vi "Entradas.vi"(11 "Class 2.lvclass":refnum<class "Class 2.lvclass">) -> (3 "Class 2.lvclass 2":refnum<class "Class 2.lvclass">)   [LabVIEW 2019, in "Class 2.lvclass"]
uses:
  Class 2.lvclass
  Class 2.lvclass/Class 2.ctl
  Datos Out.vi
  Datos In.vi
panel:
  out "current time":u32
  out "current time 2":u32
  in  "PRUEBA DE CONTACTOS":string(combo)
  in  "PRUEBA DE DISTANCIA":string(combo)
  in  "PRUEBA DE TENSION":string(combo)
  in  "ENTRADAS.HOME C2":bool
  in  "ENTRADAS.PIEZA EN EL NIDO":bool
  in  "ENTRADAS.SMAC TOMA DE MUESTRA":bool
  in  "ENTRADAS.SMAC APROXIMACION":bool
  in  "ENTRADAS.SMAC AVANCE SEGURO":bool
  in  "ENTRADAS.SMAC HOME":bool
  in  "ENTRADAS.AVANCE C2":bool
  in  "ENTRADAS.AVANCE C1":bool
  in  "ENTRADAS.HOME C1":bool
  in  "ENTRADAS.BIMANUAL 2":bool
  in  "ENTRADAS.BIMANUAL 1":bool
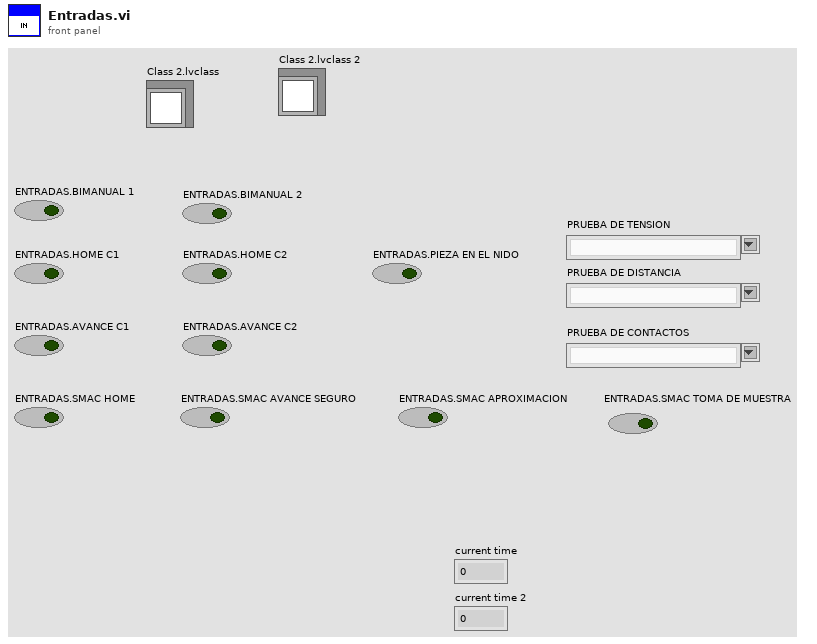
[diagram p1: front panel]
types:
  T1 = cluster{"Test":bool, "CILINDRO _1":bool, "CILINDRO _2":bool, "SMAC_RETORNANDO":bool, "SMAC_AVANZANDO":bool, "MANUAL":bool, "EST_1":bool, "EST_2":bool, "EST_3":bool, "MOVER A ORIGEN":bool, "RESET":bool, "PARO":bool, "INICIO":bool, "DATA_CONTROL":cluster{"ESTACION_1":cluster{"ACEPTADA":bool, "MAXIMO":dbl, "MINIMO":dbl, "LECTURA":dbl}, "ESTACION_2":cluster{"ACEPTADA":bool, "MAXIMO":dbl, "MINIMO":dbl, "LECTURA":dbl}, "ESTACION_3":cluster{"ACEPTADA":bool, "MAXIMO":dbl, "MINIMO":dbl, "LECTURA":dbl}}, "INGENIERIA O PROCESO":bool}
  T2 = cluster{"SALIDAS.CILINDRO 1":bool, "SALIDAS.CILINDRO 2":bool, "SALIDAS.SEMAC RETORNANDO":bool, "SALIDAS.SAMAC AVANZANDO":bool, "Auto(off)/Manual(on)":bool, "HOME_CILINDRO_1":bool, "HOME_CILINDRO_2":bool, "AVANCE_CILINDRO_1":bool, "AVANCE_CILINDRO_2":bool, "PIEZA_EN_NIDO":bool, "BIMANUAL 2":bool, "BIMANUAL1":bool, "SIN CAMBIOS":bool, "CON  CAMBIOS":bool, "TESTER":bool, "MAQUINA EN ORIGEN":bool, "FALLA PRESENTE":bool}
  T3 = cluster{"DATO GAP":string, "DATO TENSION":string, "mensajes usuario":string}
  T4 = cluster{"Numeric":dbl, "VALOR DE DISTANCIA":dbl, "VALOR DE TENSION":dbl}
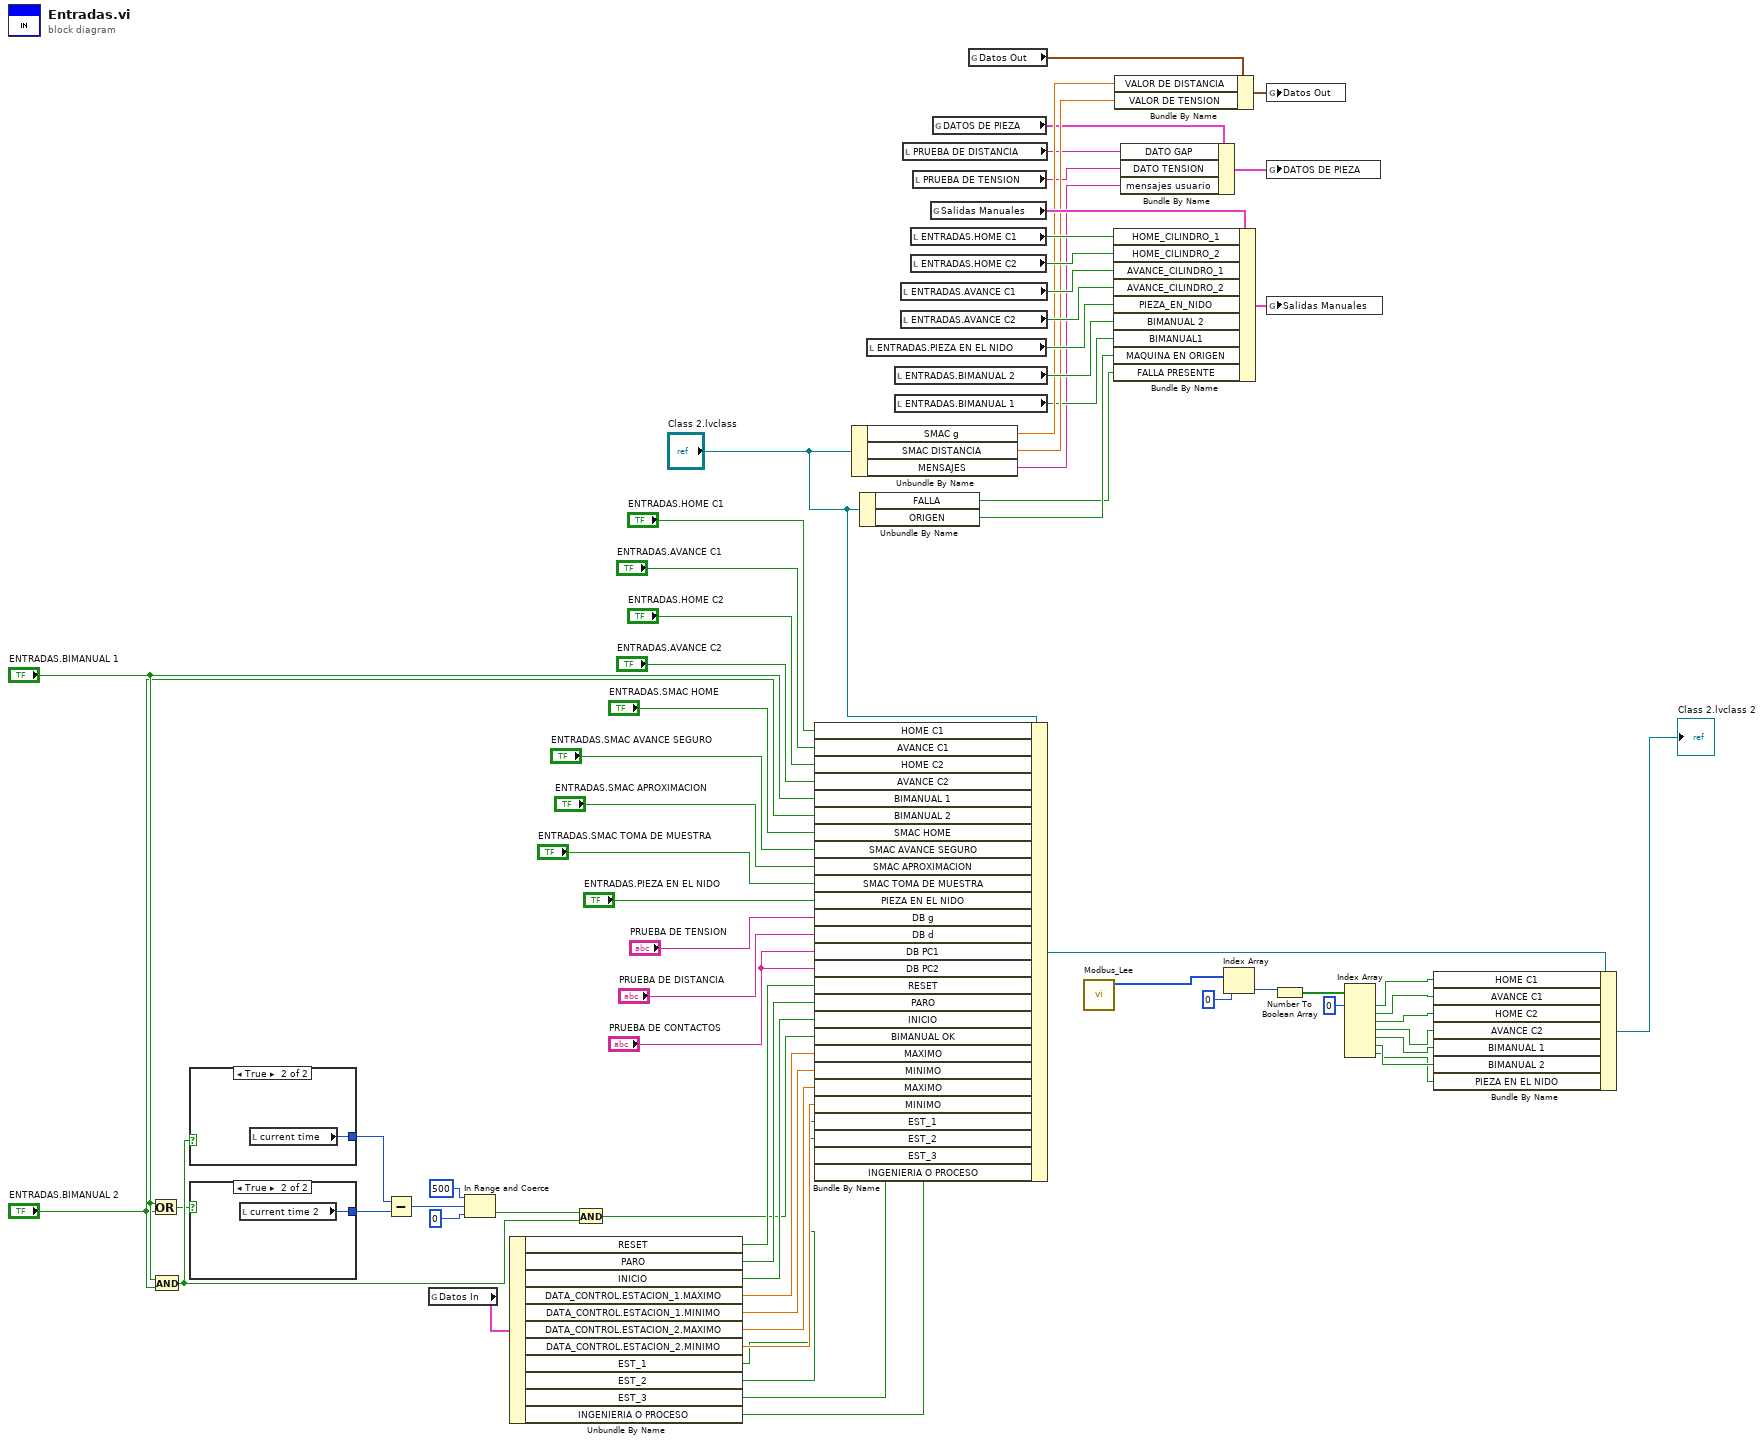
[diagram p0: block diagram]
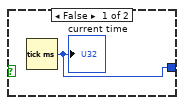
[diagram p2: hidden frame]
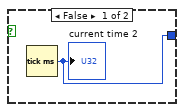
[diagram p3: hidden frame]
diagram:
  n1 = Or(x="ENTRADAS.BIMANUAL 1", y="ENTRADAS.BIMANUAL 2") -> (x .or. y?=w29:bool)
  n2 = And(x="ENTRADAS.BIMANUAL 1", y="ENTRADAS.BIMANUAL 2") -> (x .and. y?=w33:bool)
  n3 = case shown="True" w33 {
    tunnel: [w71 w72] -> w28
    frame False {
      n4 = Tick Count (ms)() -> (millisecond timer value=w71:u32)
      "current time" <- w71
    }
    frame True {
      n5 = local read "current time"() -> (w72:u32)
    }
  }
  n6 = case shown="True" w29 {
    tunnel: [w73 w74] -> w27
    frame False {
      n7 = Tick Count (ms)() -> (millisecond timer value=w73:u32)
      "current time 2" <- w73
    }
    frame True {
      n8 = local read "current time 2"() -> (w74:u32)
    }
  }
  n9 = Subtract(x=w28, y=w27) -> (x-y=w30:u32)
  n10 = global read "Datos In.vi" "Datos In"() -> (w46:T1)
  n11 = In Range and Coerce(upper limit=u32 500, x=w30, lower limit=u32 0) -> (In Range?=w32:bool)  [unwired: 1 out]
  n12 = Unbundle By Name(w46) -> ("RESET"=w45:bool, "PARO"=w44:bool, "INICIO"=w34:bool, "DATA_CONTROL.ESTACION_1.MAXIMO"=w22:dbl, "DATA_CONTROL.ESTACION_1.MINIMO"=w21:dbl, "DATA_CONTROL.ESTACION_2.MAXIMO"=w20:dbl, "DATA_CONTROL.ESTACION_2.MINIMO"=w19:dbl, "EST_1"=w4:bool, "EST_2"=w3:bool, "EST_3"=w2:bool, "INGENIERIA O PROCESO"=w1:bool)
  n13 = And(x=w32, y=w33) -> (x .and. y?=w25:bool)
  n14 = Bundle By Name(cluster="Class 2.lvclass", "HOME C1"="ENTRADAS.HOME C1", "AVANCE C1"="ENTRADAS.AVANCE C1", "HOME C2"="ENTRADAS.HOME C2", "AVANCE C2"="ENTRADAS.AVANCE C2", "BIMANUAL 1"="ENTRADAS.BIMANUAL 1", "BIMANUAL 2"="ENTRADAS.BIMANUAL 2", "SMAC HOME"="ENTRADAS.SMAC HOME", "SMAC AVANCE SEGURO"="ENTRADAS.SMAC AVANCE SEGURO", "SMAC APROXIMACION"="ENTRADAS.SMAC APROXIMACION", "SMAC TOMA DE MUESTRA"="ENTRADAS.SMAC TOMA DE MUESTRA", "PIEZA EN EL NIDO"="ENTRADAS.PIEZA EN EL NIDO", "DB g"="PRUEBA DE TENSION", "DB d"="PRUEBA DE DISTANCIA", "DB PC1"="PRUEBA DE CONTACTOS", "DB PC2"="PRUEBA DE CONTACTOS", "RESET"=w45, "PARO"=w44, "INICIO"=w34, "BIMANUAL OK"=w25, "MAXIMO"=w22, "MINIMO"=w21, "MAXIMO"=w20, "MINIMO"=w19, "EST_1"=w4, "EST_2"=w3, "EST_3"=w2, "INGENIERIA O PROCESO"=w1) -> (w13:refnum<class "Class 2.lvclass">)
  n15 = Unbundle By Name("Class 2.lvclass") -> ("SMAC g"=w48:dbl, "SMAC DISTANCIA"=w47:dbl, "MENSAJES"=w35:string)
  n16 = Unbundle By Name("Class 2.lvclass") -> ("FALLA"=w40:bool, "ORIGEN"=w41:bool)
  n17 = local read "ENTRADAS.PIEZA EN EL NIDO"() -> (w52:bool)
  n18 = local read "ENTRADAS.BIMANUAL 2"() -> (w51:bool)
  n19 = local read "ENTRADAS.BIMANUAL 1"() -> (w43:bool)
  n20 = local read "ENTRADAS.AVANCE C1"() -> (w54:bool)
  n21 = local read "ENTRADAS.AVANCE C2"() -> (w53:bool)
  n22 = local read "PRUEBA DE DISTANCIA"() -> (w37:string)
  n23 = local read "ENTRADAS.HOME C1"() -> (w56:bool)
  n24 = local read "ENTRADAS.HOME C2"() -> (w55:bool)
  n25 = local read "PRUEBA DE TENSION"() -> (w36:string)
  n26 = global read "Datos Out.vi" "Salidas Manuales"() -> (w58:T2)
  n27 = global read "Datos Out.vi" "DATOS DE PIEZA"() -> (w39:T3)
  n28 = global read "Datos Out.vi" "Datos Out"() -> (w50:T4)
  n29 = call "Modbus_Lee.vi"() -> ("register values"=w18:u16[])  [unwired: 11 in]
  n30 = Bundle By Name(cluster=w58, "HOME_CILINDRO_1"=w56, "HOME_CILINDRO_2"=w55, "AVANCE_CILINDRO_1"=w54, "AVANCE_CILINDRO_2"=w53, "PIEZA_EN_NIDO"=w52, "BIMANUAL 2"=w51, "BIMANUAL1"=w43, "MAQUINA EN ORIGEN"=w41, "FALLA PRESENTE"=w40) -> (w57:T2)
  n31 = Bundle By Name(cluster=w50, "VALOR DE DISTANCIA"=w48, "VALOR DE TENSION"=w47) -> (w49:T4)
  n32 = Bundle By Name(cluster=w39, "DATO GAP"=w37, "DATO TENSION"=w36, "mensajes usuario"=w35) -> (w38:T3)
  n33 = Index Array(array=w18, index=0) -> (element=w16:u16)
  n34 = global write "Datos Out.vi" "Datos Out"(w49) -> ()
  n35 = global write "Datos Out.vi" "DATOS DE PIEZA"(w38) -> ()
  n36 = global write "Datos Out.vi" "Salidas Manuales"(w57) -> ()
  n37 = Number To Boolean Array(number=w16) -> (Boolean array=w15:bool[])
  n38 = Index Array(array=w15, index #1=0 ("index")) -> (element #1=w11:bool, element #2=w10:bool, element #3=w9:bool, element #4=w8:bool, element #5=w7:bool, element #6=w6:bool, element #7=w5:bool)  [unwired: 6 in]
  n39 = Bundle By Name(cluster=w13, "HOME C1"=w11, "AVANCE C1"=w10, "HOME C2"=w9, "AVANCE C2"=w8, "BIMANUAL 1"=w7, "BIMANUAL 2"=w6, "PIEZA EN EL NIDO"=w5) -> (→"Class 2.lvclass 2":refnum<class "Class 2.lvclass">)
